vi "Read UI VI Reference.vi"(11 "Flex UI in":refnum<class "Flex UI.lvclass">) -> (2 "UI VI Reference":refnum<vi>, 3 "Flex UI out":refnum<class "Flex UI.lvclass">)   [LabVIEW 2016, in "Flex UI.lvclass"]
uses:
  Flex UI.lvclass
  Flex UI.lvclass/Flex UI.ctl
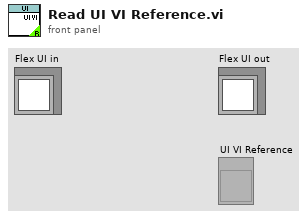
[diagram p1: front panel]
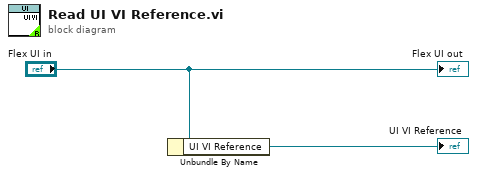
[diagram p0: block diagram]
diagram:
  n1 = Unbundle By Name("Flex UI in") -> ("UI VI Reference"=→"UI VI Reference":refnum<vi>)
  "Flex UI out" <- "Flex UI in"
